vi "Total Noise Difference.vi"(10 "Array 2":u8[][](array[numeric]), 11 "Array":u8[][](array[numeric])) -> (3 "Numeric":u8)   [LabVIEW 2016]
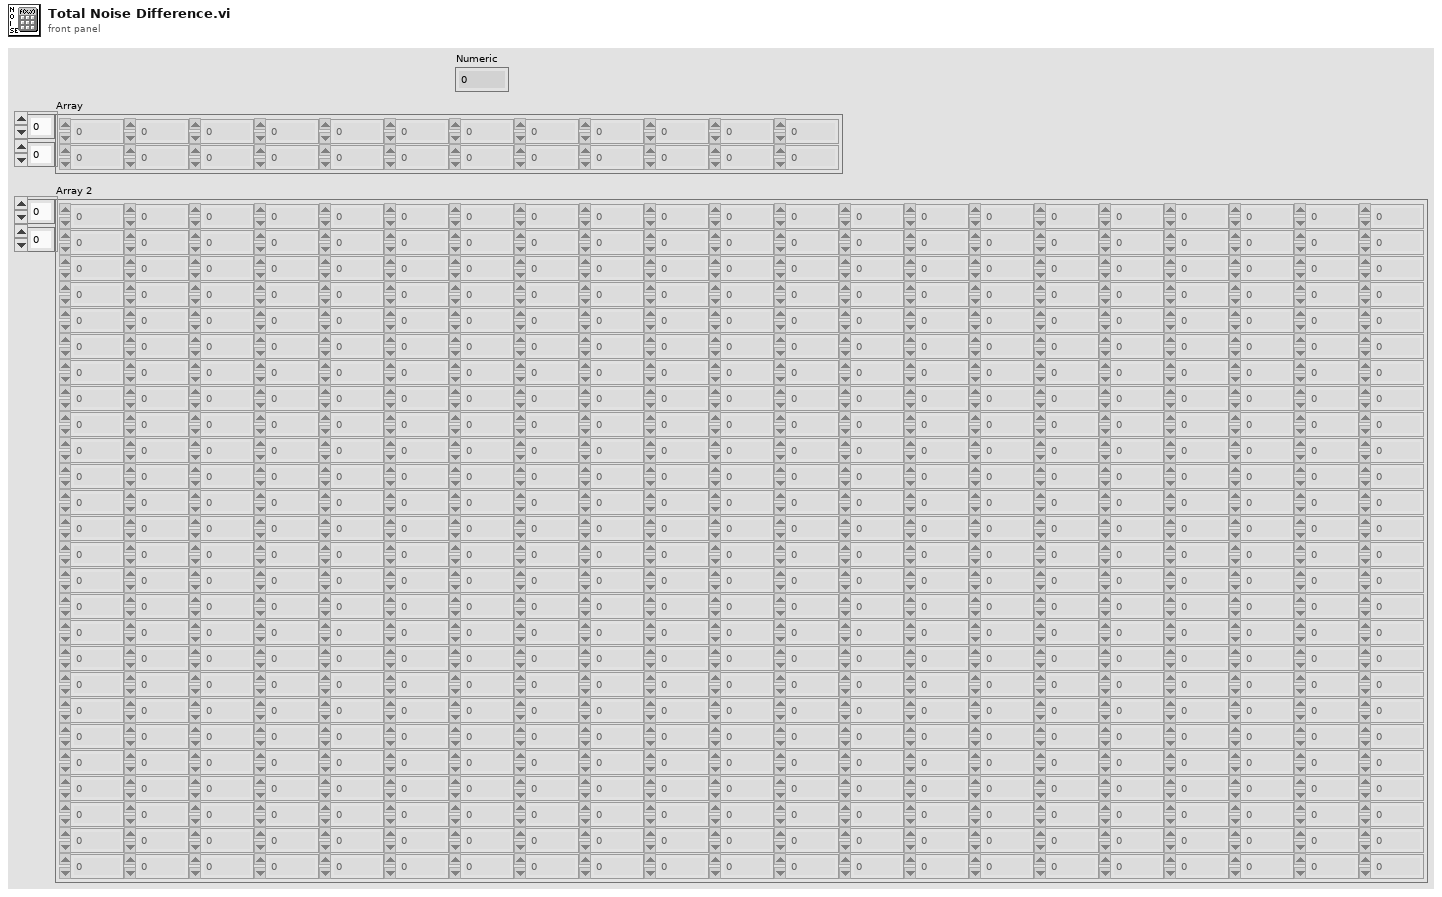
[diagram p1: front panel]
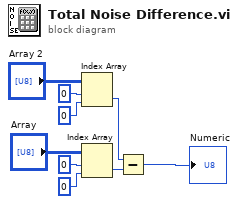
[diagram p0: block diagram]
diagram:
  n1 = Index Array(array="Array 2", index (row)=0, index (col)=0 ("disabled index (col)")) -> (element=w4:u8)
  n2 = Index Array(array="Array", index (row)=0, index (col)=0 ("disabled index (col)")) -> (element=w9:u8)
  n3 = Subtract(x=w4, y=w9) -> (x-y=→"Numeric":u8)
